vi "Inject Attribute List.vi"(6 "Attributes Ref":refnum<data-value>, 8 "error in (no error)":errorcluster, 11 "Stop Pre-Soak in":refnum<class "Stop Pre-Soak.lvclass">) -> (0 "error out":errorcluster, 3 "Stop Pre-Soak out":refnum<class "Stop Pre-Soak.lvclass">)   [LabVIEW 2019, in "Stop Pre-Soak.lvclass"]
uses:
  <vilib>/gpm_packages/@cs/Car-wash/Source/Process Steps/Stop Pre-Soak/Stop Pre-Soak.lvclass
  <vilib>/gpm_packages/@cs/lookup-table/Source/LookupTable/LookupTable.lvclass
  <vilib>/gpm_packages/@cs/lookup-table/Source/LookupTable/LookupTable.lvclass/LookupTable.ctl
  <vilib>/gpm_packages/@cs/Car-wash/Source/Process Steps/Stop Pre-Soak/Stop Pre-Soak.lvclass/Stop Pre-Soak.ctl
  24e8c90e-f533-4af5-b895-9daf0d109a1d.vi
  <vilib>/gpm_packages/@cs/lookup-table/Source/LookupTable/Read Table Reference.vi
  24e8c90e-f533-4af5-b895-9daf0d109a1d.vi/22ebf123-5a71-454c-85f5-12e9b6a84ed0.vi
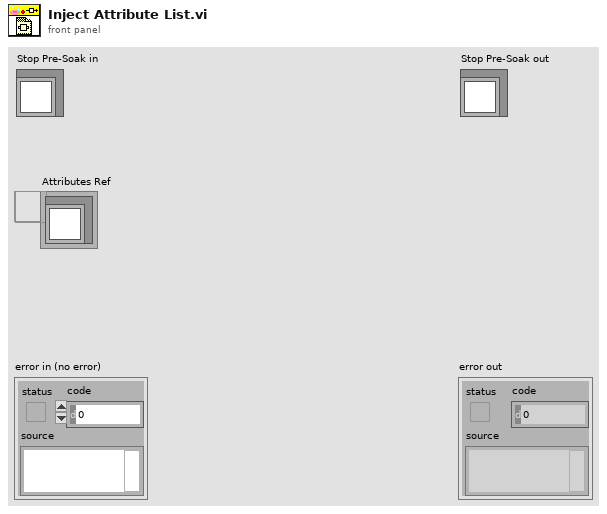
[diagram p1: front panel]
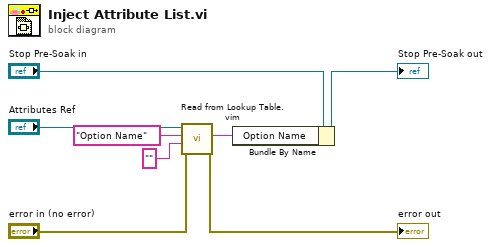
[diagram p0: block diagram]
diagram:
  n1 = call "Read from Lookup Table.vim"("error in (no error)"="error in (no error)", "Type"="", "Item Name"="Option Name", "LookupTable Reference"="Attributes Ref") -> ("error out"=→"error out":errorcluster, "Value"=w6:string)  [unwired: 4 in, 2 out]
  n2 = Bundle By Name(cluster="Stop Pre-Soak in", "Option Name"=w6) -> (→"Stop Pre-Soak out":refnum<class "Stop Pre-Soak.lvclass">)
